vi "Adding Channels.vi"() -> ()   [LabVIEW 2015]
uses:
  <instrlib>/niSwitch/niSwitch.LLB/niSwitch Topologies.ctl
panel:
  in  "Channels":i32[](listbox)
  out "error out":errorcluster
  in  "Switch Model":string(combo)
  in  "Topology":string(combo)
  in  "Remove All":bool
  in  "Add All":bool
  in  "stop":bool
  in  "Topology Names":T1="2503/2-Wire 24x1 Mux" caption="topology name"
  in  "Selectable Channels":i32[](listbox)
  in  "Remove Channels":bool
  in  "Add Channels":bool
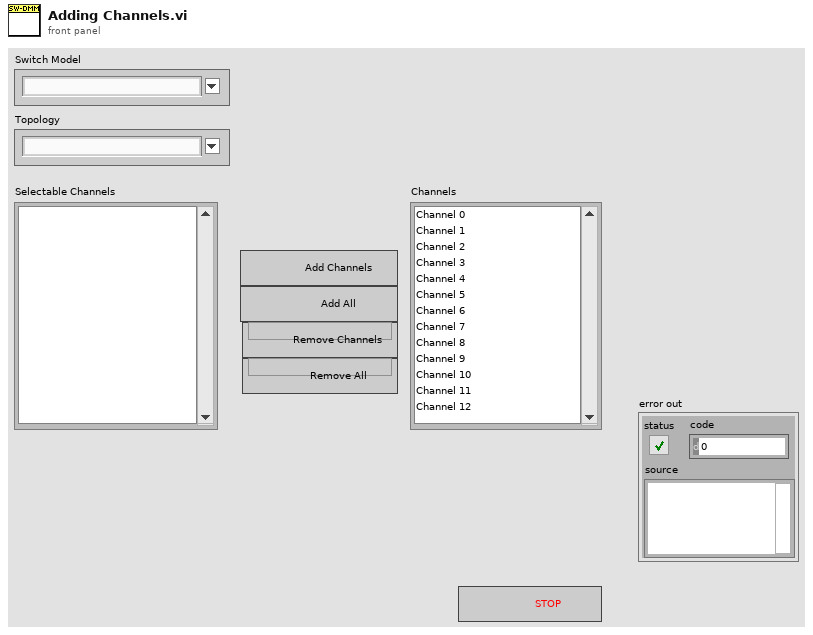
[diagram p1: front panel]
types:
  T1 = typedef "niSwitch Topologies.ctl" = string
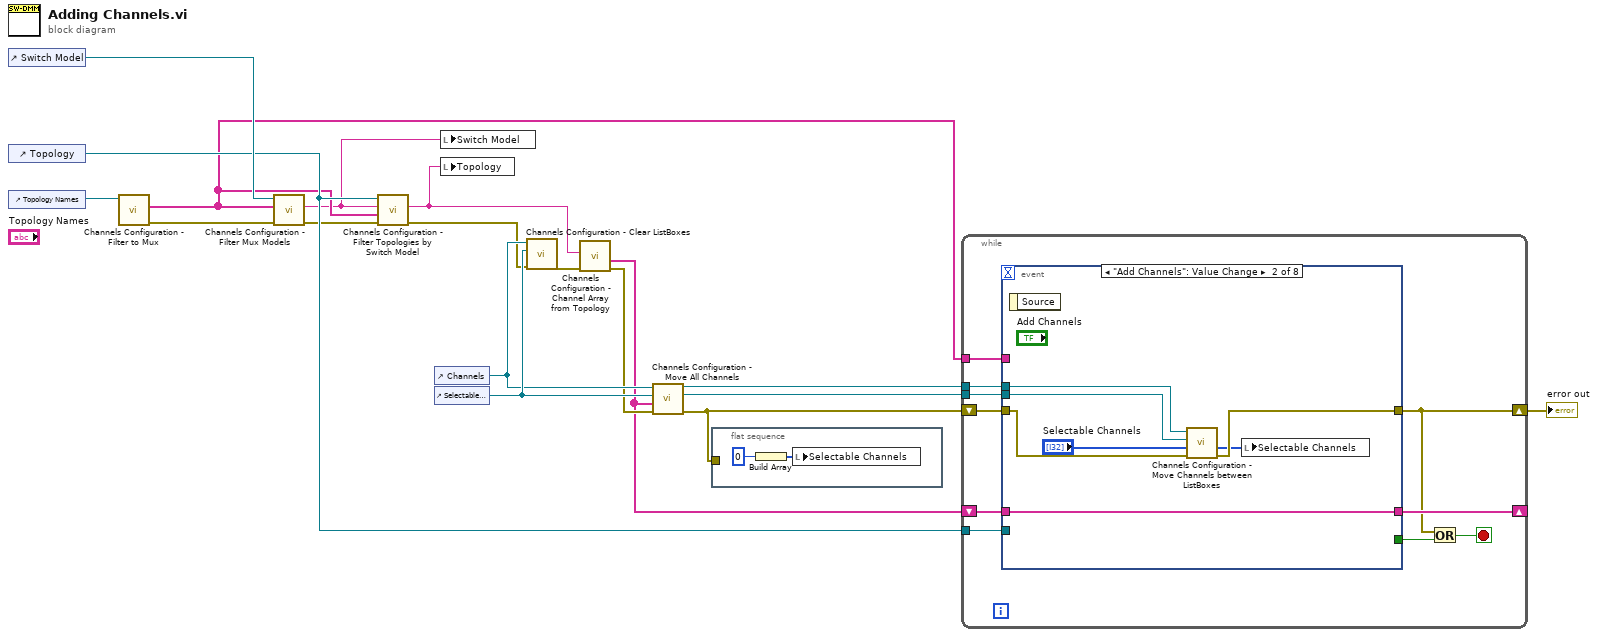
[diagram p0: block diagram]
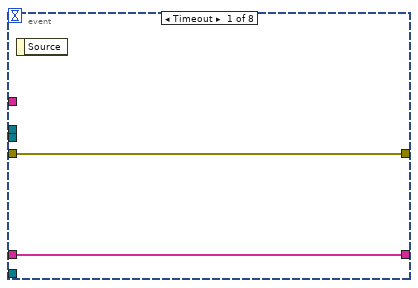
[diagram p2: hidden frame]
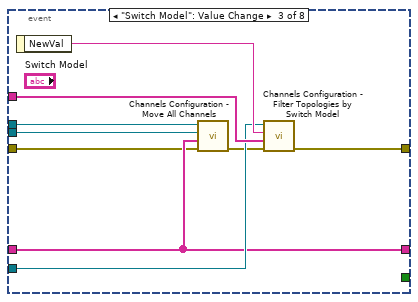
[diagram p3: hidden frame]
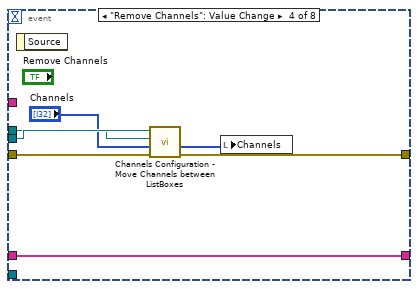
[diagram p4: hidden frame]
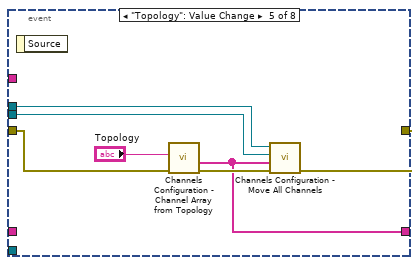
[diagram p5: hidden frame]
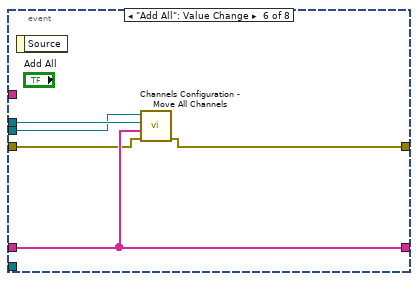
[diagram p6: hidden frame]
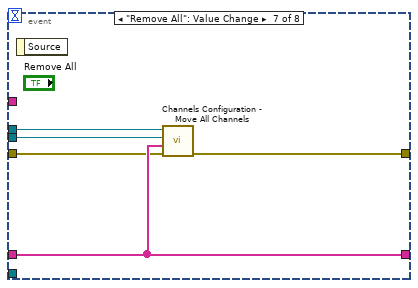
[diagram p7: hidden frame]
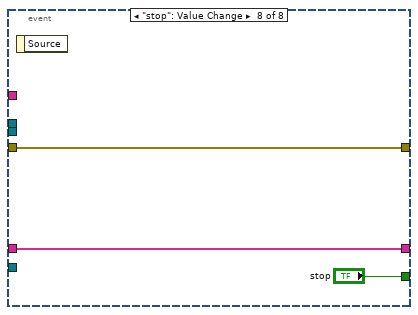
[diagram p8: hidden frame]
diagram:
  n1 = control-ref of="Switch Model"() -> (w14:refnum<vi>)
  n2 = control-ref of="Topology"() -> (w8:refnum<vi>)
  n3 = control-ref of="Topology Names"() -> (w15:refnum<vi>)
  n4 = call "Channels Configuration - Filter to Mux.vi"("ComboBox in"=w15) -> ("error out"=w7:errorcluster, "Mux List"=w4:string[])  [unwired: 9 in]
  n5 = call "Channels Configuration - Filter Mux Models.vi"("error in (no error)"=w7, "Mux List"=w4, "ComboBox in"=w14) -> ("error out"=w6:errorcluster, "First Mux Model"=w3:string)  [unwired: 7 in]
  n6 = call "Channels Configuration - Filter Topologies by Switch Model.vi"("error in (no error)"=w6, "Mux List"=w4, "Switch Model"=w3, "Topology Control Ref In"=w8) -> ("error out"=w9:errorcluster, "First Topology from List"=w2:string)  [unwired: 6 in]
  n7 = control-ref of="Channels"() -> (w12:refnum<vi>)
  n8 = control-ref of="Selectable Channels"() -> (w18:refnum<vi>)
  n9 = local write "Switch Model"(w3) -> ()
  n10 = local write "Topology"(w2) -> ()
  n11 = call "Channels Configuration - Clear ListBoxes.vi"("error in (no error)"=w9, "ListBox 2 Ref In"=w18, "ListBox 1 Ref In"=w12) -> ("error out"=w11:errorcluster)  [unwired: 6 in, 2 out]
  n12 = call "Channels Configuration - Channel Array from Topology.vi"("error in (no error)"=w11, "Selected Mux Topology"=w2) -> ("error out"=w10:errorcluster, "Channel Array Out"=w1:string[])  [unwired: 8 in]
  n13 = call "Channels Configuration - Move All Channels.vi"("error in (no error)"=w10, "All Items"=w1, "Destiny Listbox Ref In"=w18, "Origin ListBox Ref In"=w12) -> ("error out"=w5:errorcluster, "Destiny ListBox Ref Out"=w17:refnum<vi>, "Origin ListBox Ref Out"=w16:refnum<vi>)  [unwired: 5 in]
  n14 = flat-sequence {
    tunnel: w5 -> [_]
    frame #0 {
      n15 = Build Array(0) -> (w20:i32[])
      n16 = local write "Selectable Channels"(w20) -> ()
    }
  }
  n17 = while {
    tunnel: w17 -> [w30]
    tunnel: w16 -> [w29]
    shift-right: [w27] -> _
    shift-left: w1 -> [w26]
    tunnel: w4 -> [w25]
    shift-right: [w24] -> w13
    shift-left: w5 -> [w28]
    tunnel: w8 -> [w21]
    stop <- w23 stop-if-true
    n18 = event shown="[1] \"Add Channels\": Value Change" {
      selector: _ -> [_ _ _ _ _ _ _ _]
      dyn-events: _ -> [_ _ _ _ _ _ _ _]
      timeout: _ -> [_ _ _ _ _ _ _ _]
      tunnel: w30 -> [_ w39 w44 w54 w60 w64 w72 _]
      tunnel: w29 -> [_ w37 w42 w53 w59 w67 w71 _]
      tunnel: w28 -> [w31 w38 w41 w52 w62 w65 w69 w74]
      tunnel: [w32 w36 w43 w55 w56 w66 w70 w75] -> w27
      tunnel: w26 -> [w32 w36 w43 w55 _ w66 w70 w75]
      tunnel: w25 -> [_ _ w48 _ _ _ _ _]
      tunnel: [w31 w34 w46 w51 w57 w63 w68 w74] -> w24
      tunnel: [_ _ _ _ _ _ _ "stop"] -> w22
      tunnel: w21 -> [_ _ w45 _ _ _ _ _]
      event Timeout {
        n19 = event-data() -> ()  [unwired: 1 in, 1 out]
      }
      event "Add Channels": Value Change {
        n20 = event-data() -> ()  [unwired: 1 in, 1 out]
        n21 = call "Channels Configuration - Move Channels between ListBoxes.vi"("error in (no error)"=w38, "ListBox Origin In"="Selectable Channels", "ListBox Origin Ref In"=w39, "ListBox Destiny Ref In"=w37) -> ("error out"=w34:errorcluster, "ListBox Out"=w33:i32[])  [unwired: 4 in, 2 out]
        n22 = local write "Selectable Channels"(w33) -> ()
      }
      event "Switch Model": Value Change {
        n23 = event-data() -> ("NewVal"=w47:string)  [unwired: 1 in]
        n24 = call "Channels Configuration - Move All Channels.vi"("error in (no error)"=w41, "All Items"=w43, "Destiny Listbox Ref In"=w44, "Origin ListBox Ref In"=w42) -> ("error out"=w40:errorcluster)  [unwired: 5 in, 2 out]
        n25 = call "Channels Configuration - Filter Topologies by Switch Model.vi"("error in (no error)"=w40, "Mux List"=w48, "Switch Model"=w47, "Topology Control Ref In"=w45) -> ("error out"=w46:errorcluster)  [unwired: 6 in, 1 out]
      }
      event "Remove Channels": Value Change {
        n26 = event-data() -> ()  [unwired: 1 in, 1 out]
        n27 = call "Channels Configuration - Move Channels between ListBoxes.vi"("error in (no error)"=w52, "ListBox Origin In"="Channels", "ListBox Origin Ref In"=w53, "ListBox Destiny Ref In"=w54) -> ("error out"=w51:errorcluster, "ListBox Out"=w49:i32[])  [unwired: 4 in, 2 out]
        n28 = local write "Channels"(w49) -> ()
      }
      event "Topology": Value Change {
        n29 = event-data() -> ()  [unwired: 1 in, 1 out]
        n30 = call "Channels Configuration - Channel Array from Topology.vi"("error in (no error)"=w62, "Selected Mux Topology"="Topology") -> ("error out"=w58:errorcluster, "Channel Array Out"=w56:string[])  [unwired: 8 in]
        n31 = call "Channels Configuration - Move All Channels.vi"("error in (no error)"=w58, "All Items"=w56, "Destiny Listbox Ref In"=w60, "Origin ListBox Ref In"=w59) -> ("error out"=w57:errorcluster)  [unwired: 5 in, 2 out]
      }
      event "Add All": Value Change {
        n32 = event-data() -> ()  [unwired: 1 in, 1 out]
        n33 = call "Channels Configuration - Move All Channels.vi"("error in (no error)"=w65, "All Items"=w66, "Destiny Listbox Ref In"=w67, "Origin ListBox Ref In"=w64) -> ("error out"=w63:errorcluster)  [unwired: 5 in, 2 out]
      }
      event "Remove All": Value Change {
        n34 = event-data() -> ()  [unwired: 1 in, 1 out]
        n35 = call "Channels Configuration - Move All Channels.vi"("error in (no error)"=w69, "All Items"=w70, "Destiny Listbox Ref In"=w72, "Origin ListBox Ref In"=w71) -> ("error out"=w68:errorcluster)  [unwired: 5 in, 2 out]
      }
      event "stop": Value Change {
        n36 = event-data() -> ()  [unwired: 1 in, 1 out]
      }
    }
    n37 = Or(x=w24, y=w22) -> (x .or. y?=w23:bool)
  }
  "error out" <- w13
